vi "Array of Variants to JSON Array.vi"(4 "LVClass Serializer":refnum<class "JSONtext LVClass Serializer.lvclass">, 5 "enable LabVIEW extensions? (T)":bool=TRUE, 6 "Pretty Print?":bool, 9 "error in (no error)":errorcluster, 11 "Array of Variants":variant[](array[variant])) -> (1 "error out":errorcluster, 3 "<JSON>":string caption="<JSON>Array")   [LabVIEW 2017, in "JSONtext.lvlib"]
doc: "Flatten an Array of Variants into a JSON Array. \n\nStrings or Arrays of strings marked with a leading <JSON> tag in their name (including inside clusters) are treated as already being valid JSON. Strings not marked as <JSON> are quoted and escaped as a JSON String."
uses:
  JSONtext.lvlib
  LVClass Serializer/JSONtext LVClass Serializer.lvclass
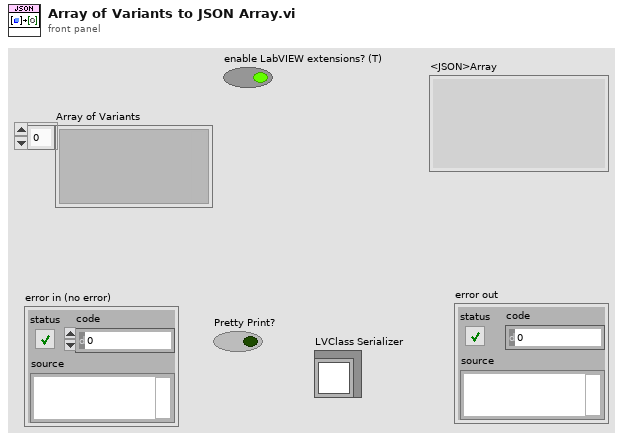
[diagram p1: front panel]
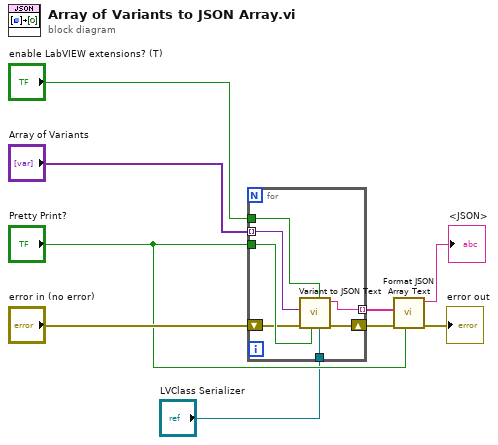
[diagram p0: block diagram]
diagram:
  n1 = for {
    tunnel: "Array of Variants" -> [w16] mode=indexing
    tunnel: "Pretty Print?" -> [w15]
    tunnel: [w11] -> w4 mode=indexing
    shift-right: [w14] -> w7
    shift-left: "error in (no error)" -> [w13]
    tunnel: "enable LabVIEW extensions? (T)" -> [w12]
    tunnel: "LVClass Serializer" -> [w10]
    n2 = call "Variant to JSON Text.vi"("LVClass Serializer"=w10, "enable LabVIEW extensions? (T)"=w12, "Pretty Print?"=w15, "error in (no error)"=w13, "Variant"=w16) -> ("error out"=w14:errorcluster, "<JSON>"=w11:string)  [unwired: 4 in, 1 out]
  }
  n3 = call "Format JSON Array Text.vi"("Pretty Print?"="Pretty Print?", "error in (no error)"=w7, "Array of JSON Text"=w4) -> ("error out"=→"error out":errorcluster, "<JSON>"=→"<JSON>":string)  [unwired: 7 in]
